vi "Append String To Path.vi"(10 "name":string, 11 "path in":path) -> (3 "appended path out":path)   [LabVIEW 2019]
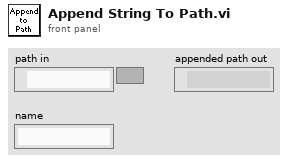
[diagram p1: front panel]
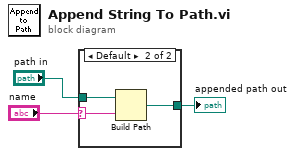
[diagram p0: block diagram]
diagram:
  n1 = case shown="Default" "name" {
    selector: "name" -> [_ w5]
    tunnel: "path in" -> [w4 w7]
    tunnel: [w4 w6] -> w2
    frame "" {
    }
    frame Default {
      n2 = Build Path(base path=w7, name or relative path=w5) -> (appended path=w6:path)
    }
  }
  "appended path out" <- w2
